vi "svl_Log View for Energy Level (WDT).vi"(7 "channel info":T1={"sensor sensitivity"=1000.0, "engineering units"=1, "dB reference"=1.0, "custom label"="EU", "weighting filter"=0, "pregain"=0.0} {"pregain" format="%.2f"; "weighting filter" items=["Linear", "A-weighting", "B-weighting", "C-weighting", "ITU-R 468-4", "Dolby", "CCITT", "C-message", "Wb", "Wc", "Wd", "We", "Wf", "Wh", "Wj", "Wk", "Wm", "AES17 20 kHz lowpass", "AES17 40 kHz lowpass", "AES17 20 kHz highpass", "AES17 40 kHz highpass"]; "dB reference" format="%^.1e"; "engineering units" items=["custom..."=0, "V"=1, "A"=21, "C"=30, "pC"=31, "s"=32, "-"=29, "Pa"=2, "N"=20, "g"=3, "m/s^2"=4, "m/s"=5, "m"=6, "mm/s"=12, "mm"=13, "micron/s"=14, "micron"=15, "in/s^2"=7, "in/s"=8, "in"=9, "mil/s"=10, "mil"=11, "rad/s^2"=16, "rad/s"=17, "rad"=18, "deg/s^2"=26, "deg/s"=27, "deg"=28, "RPM"=22, "cycle/s^2"=23, "Hz"=24, "cycle"=25, "strain"=19]; "sensor sensitivity" format="%#_5f"}, 8 "error in (no error)":errorcluster, 9 "view mode":enum16{"Power", "Amplitude"}(ring), 10 "dB On (T)":bool=TRUE, 11 "scaledSignal":waveform(dbl)={"t0"=timestamp(0 s since 1904-01-01), "dt"=0.0, "Y"=[]}) -> (0 "error out":errorcluster, 2 "unit label":string, 3 "scaledSignal":waveform(dbl))   [LabVIEW 2017]
uses:
  <vilib>/addons/_NISVFA/_Shared subVIs/Controls/svc_Channel Info.ctl
  <vilib>/addons/_NISVFA/_Shared subVIs/Controls/svc_Engineering Units Text Ring.ctl
  <vilib>/addons/_NISVFA/_Shared subVIs/Controls/svc_Weighting Filter Text Ring.ctl
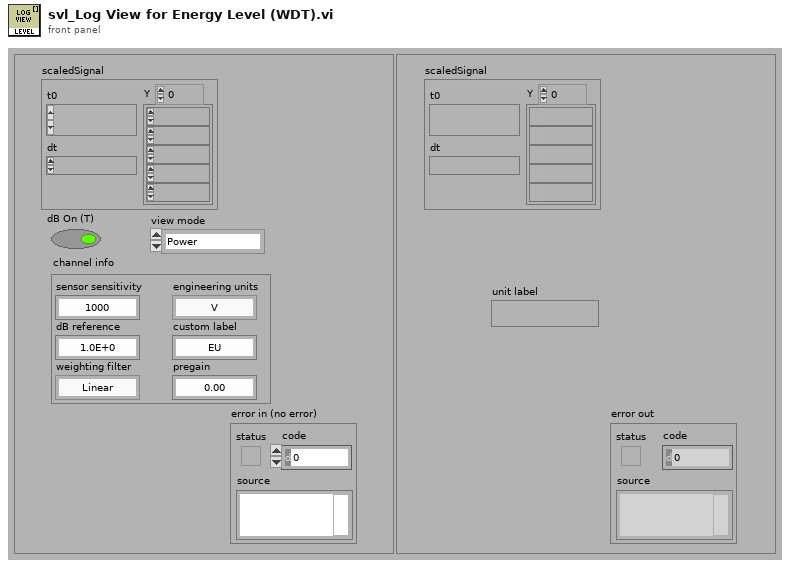
[diagram p1: front panel]
types:
  T1 = typedef "svc_Channel Info.ctl" = cluster{"sensor sensitivity":dbl, "engineering units":T2, "dB reference":dbl, "custom label":string, "weighting filter":T3, "pregain":dbl}
  T2 = typedef "svc_Engineering Units Text Ring.ctl" = u16
  T3 = typedef "svc_Weighting Filter Text Ring.ctl" = u16
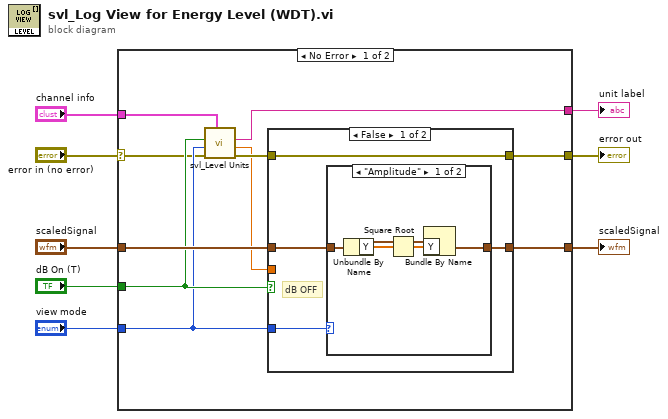
[diagram p0: block diagram]
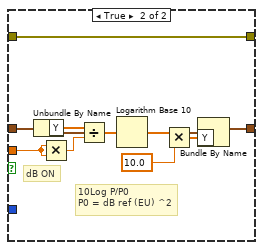
[diagram p3: hidden frame]
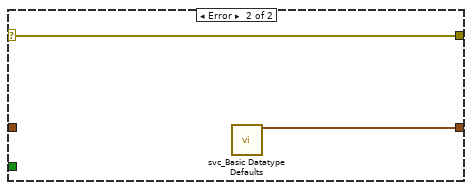
[diagram p4: hidden frame]
diagram:
  n1 = case shown="No Error" "error in (no error)" {
    selector: "error in (no error)" -> [w9 w38]
    tunnel: [w18 w38] -> w8
    tunnel: "scaledSignal" -> [w17 _]
    tunnel: [w16 w39] -> w6
    tunnel: "dB On (T)" -> [w15 _]
    tunnel: "view mode" -> [w14 _]
    tunnel: [w11 _] -> w3
    tunnel: "channel info" -> [w10 _]
    frame No Error {
      n2 = call <vilib>:"svl_Level Units.vi"("channel info"=w10, "error in (no error)"=w9, "view mode"=w14, "dB On (T)"=w15) -> ("error out"=w13:errorcluster, "dB reference [EU]"=w12:dbl, "unit label"=w11:string)  [unwired: 5 in]
      n3 = case shown="False" w15 {
        tunnel: [w22 w32] -> w16
        tunnel: w13 -> [w21 w37]
        tunnel: [w21 w37] -> w18
        tunnel: w17 -> [w19 w30]
        tunnel: w14 -> [w20 _]
        tunnel: w12 -> [_ w28]
        frame False {
          # "dB OFF"
          n4 = case shown="\"Amplitude\"" w20 {
            tunnel: [w23 w27] -> w22
            tunnel: w19 -> [w24 w27]
            frame "Amplitude" {
              n5 = Unbundle By Name(w24) -> ("Y"=w26:dbl[])
              n6 = Square Root(x=w26) -> (sqrt(x)=w25:dbl[])
              n7 = Bundle By Name(cluster=w24, "Y"=w25) -> (w23:waveform(dbl))
            }
            frame "Power", Default {
            }
          }
        }
        frame True {
          # "10Log P/P0\nP0 = dB ref (EU) ^2"
          # "dB ON"
          n8 = Unbundle By Name(w30) -> ("Y"=w33:dbl[])
          n9 = Multiply(x=w28, y=w28) -> (x*y=w29:dbl)
          n10 = Divide(x=w33, y=w29) -> (x/y=w34:dbl[])
          n11 = Logarithm Base 10(1:w34) -> (0:w35:dbl[])
          n12 = Multiply(x=w35, y=10.0) -> (x*y=w31:dbl[])
          n13 = Bundle By Name(cluster=w30, "Y"=w31) -> (w32:waveform(dbl))
        }
      }
    }
    frame Error {
      n14 = call <vilib>:"svc_Basic Datatype Defaults.vi"() -> ("empty waveform"=w39:waveform(dbl))  [unwired: 7 in, 12 out]
    }
  }
  "unit label" <- w3
  "scaledSignal" <- w6
  "error out" <- w8
